vi "NumberDateTimeToNow.vi"(9 "StartTime":string, 11 "StartDate":string) -> (2 "Hours":string)   [LabVIEW 2012]
uses:
  <vilib>/Utility/miscctls.llb/LVDateTimeRec.ctl
panel:
  in  "date time rec":T1
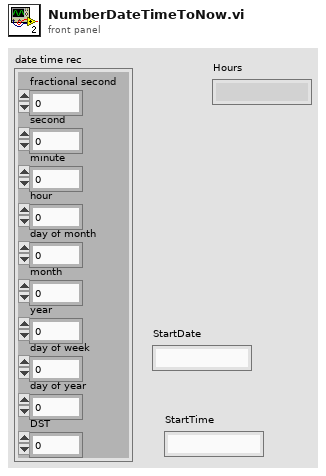
[diagram p1: front panel]
types:
  T1 = typedef "LVDateTimeRec.ctl" = cluster{"fractional second":dbl, "second":i32, "minute":i32, "hour":i32, "day of month":i32, "month":i32, "year":i32, "day of week":i32, "day of year":i32, "DST":i32}
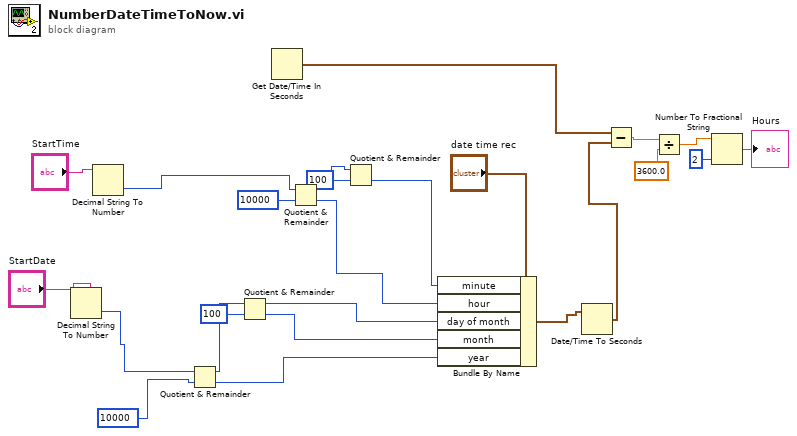
[diagram p0: block diagram]
diagram:
  n1 = Decimal String To Number(string="StartDate") -> (number=w4:i32)  [unwired: 2 in, 1 out]
  n2 = Decimal String To Number(string="StartTime") -> (number=w7:i32)  [unwired: 2 in, 1 out]
  n3 = Quotient & Remainder(x=w4, y=10000) -> (x-y*floor(x/y)=w18:i32, floor(x/y)=w19:i32)
  n4 = Quotient & Remainder(x=w18, y=100) -> (x-y*floor(x/y)=w15:i32, floor(x/y)=w16:i32)
  n5 = Get Date/Time In Seconds() -> (seconds since 1Jan1904=w9:timestamp)
  n6 = Quotient & Remainder(x=w7, y=10000) -> (x-y*floor(x/y)=w12:i32, floor(x/y)=w13:i32)
  n7 = Quotient & Remainder(x=w12, y=100) -> (floor(x/y)=w10:i32)  [unwired: 1 out]
  n8 = Bundle By Name(cluster="date time rec", "minute"=w10, "hour"=w13, "day of month"=w15, "month"=w16, "year"=w19) -> (w23:T1)
  n9 = Date/Time To Seconds(2:w23) -> (0:w8:timestamp)  [unwired: 1 in]
  n10 = Subtract(x=w9, y=w8) -> (x-y=w22:dbl)
  n11 = Divide(x=w22, y=3600.0) -> (x/y=w3:dbl)
  n12 = Number To Fractional String(number=w3, precision (6)=i16 2) -> (F-format string=→"Hours":string)  [unwired: 2 in]
